vi "Plotter_Plot_Core.vi"(7 "Plot Parameters":T1[](array[typedef]), 8 "error in (no error)":errorcluster, 9 "Refresh interval (ms)":u32, 10 "Commands":T2, 11 "XY Graph":refnum<vi>) -> (0 "error out":errorcluster)   [LabVIEW 2017]
uses:
  Controls/Plotter_UI_Plot_Commands.ctl
  Controls/Plotter_Plot_Parameter_and_Timestamp.ctl
  Controls/Plotter_Plot.ctl
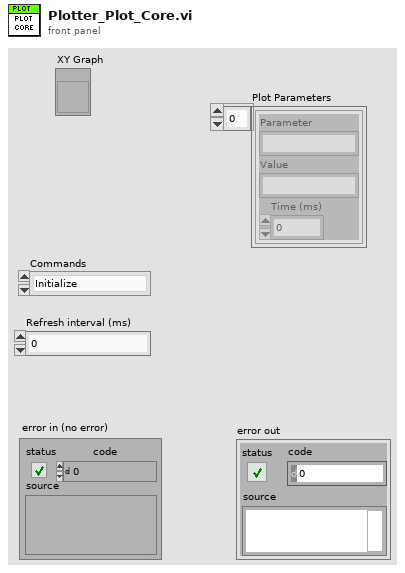
[diagram p1: front panel]
types:
  T1 = typedef "Plotter_Plot_Parameter_and_Timestamp.ctl" = cluster{"Parameter":string, "Value":string, "Time (ms)":u32}
  T2 = typedef "Plotter_UI_Plot_Commands.ctl" = enum16{"Initialize", "Update", "Clear"}
  T3 = typedef "Plotter_Plot.ctl" = cluster{"Time (ms)":dbl[], "Values":dbl[]}
  T4 = cluster{"Parameter name":string, "Samples":dbl[], "Time (ms)":dbl[]}[]
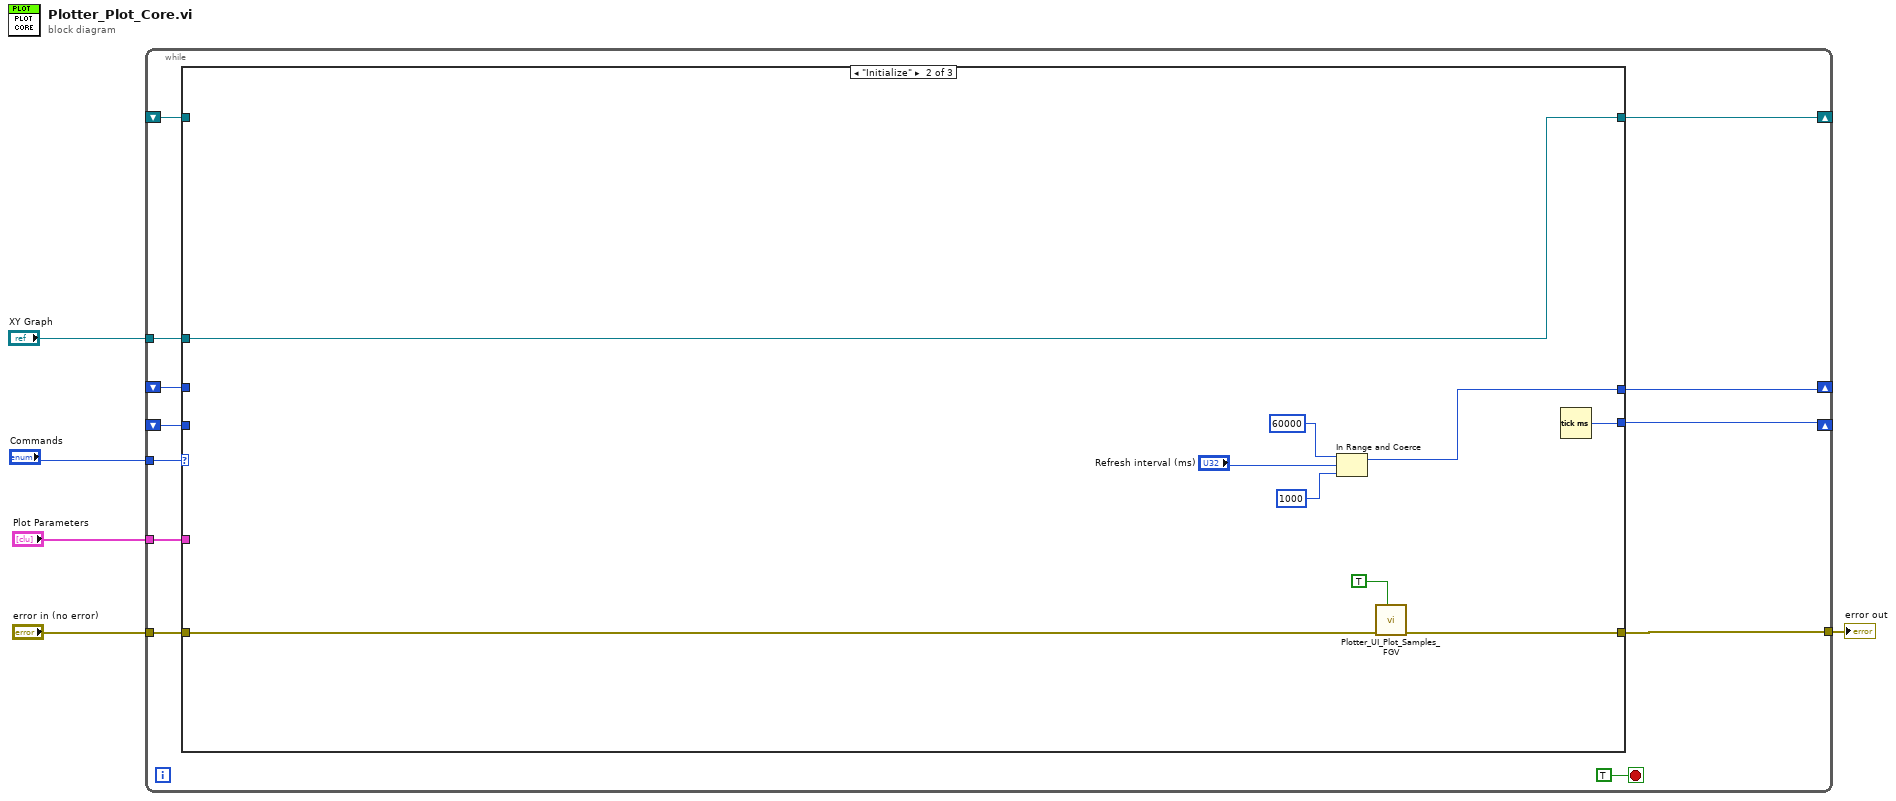
[diagram p0: block diagram]
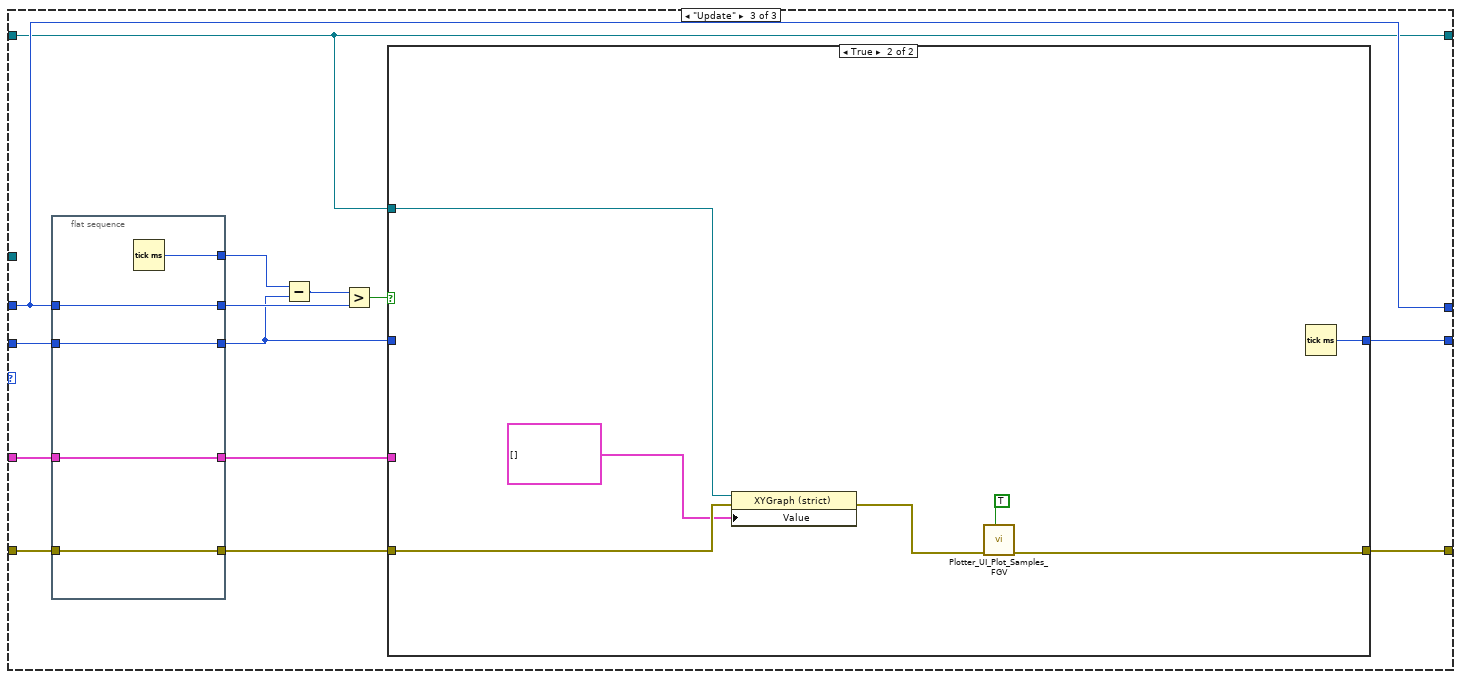
[diagram p3: hidden frame]
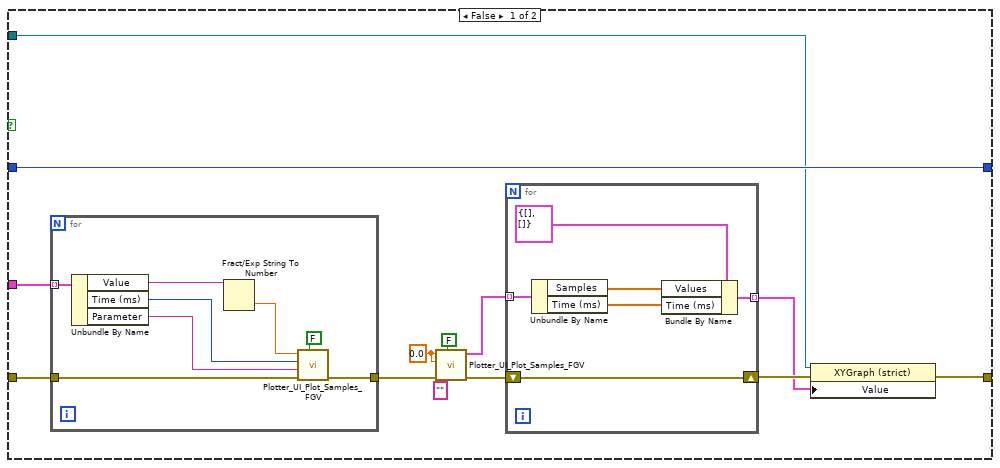
[diagram p4: hidden frame]
diagram:
  n1 = while {
    tunnel: "XY Graph" -> [w15]
    tunnel: "error in (no error)" -> [w12]
    tunnel: "Commands" -> [w16]
    shift-right: [w14] -> _
    shift-left: _ -> [w13]
    tunnel: [w11] -> w1
    shift-right: [w10] -> _
    shift-left: _ -> [w8]
    shift-right: [w9] -> _
    shift-left: _ -> [w7]
    tunnel: "Plot Parameters" -> [w6]
    stop <- TRUE stop-if-true
    n2 = case shown="\"Initialize\"" w16 {
      tunnel: w15 -> [_ w30 _]
      tunnel: [w21 w30 w31] -> w14
      tunnel: w13 -> [w21 _ w31]
      tunnel: w12 -> [w20 w24 w44]
      tunnel: [w20 w23 w34] -> w11
      tunnel: [w19 w25 w39] -> w10
      tunnel: [w18 w29 w37] -> w9
      tunnel: w8 -> [w19 _ w39]
      tunnel: w7 -> [w18 _ w43]
      tunnel: w6 -> [_ _ w33]
      frame Default {
      }
      frame "Initialize" {
        n3 = In Range and Coerce(upper limit=u32 60000, x="Refresh interval (ms)", lower limit=u32 1000) -> (coerced(x)=w25:u32)  [unwired: 1 out]
        n4 = call "Plotter_UI_Plot_Samples_FGV.vi"("Initialize ?"=TRUE, "error in (no error)"=w24) -> ("error out"=w23:errorcluster)  [unwired: 8 in, 1 out]
        n5 = Tick Count (ms)() -> (millisecond timer value=w29:u32)
      }
      frame "Update" {
        n6 = flat-sequence {
          tunnel: w44 -> [w83]
          tunnel: [w83] -> w35
          tunnel: w43 -> [w82]
          tunnel: [w82] -> w36
          tunnel: [w81] -> w42
          tunnel: w39 -> [w80]
          tunnel: [w80] -> w40
          tunnel: w33 -> [w79]
          tunnel: [w79] -> w32
          frame #0 {
            n7 = Tick Count (ms)() -> (millisecond timer value=w81:u32)
          }
        }
        n8 = Subtract(x=w42, y=w36) -> (x-y=w41:u32)
        n9 = Greater?(x=w41, y=w40) -> (0:w38:bool)
        n10 = case shown="True" w38 {
          tunnel: [w57 w78] -> w37
          tunnel: w36 -> [w57 _]
          tunnel: w35 -> [w56 w77]
          tunnel: [w47 w73] -> w34
          tunnel: w32 -> [w55 _]
          tunnel: w31 -> [w46 w76]
          frame False {
            w52 = 0.0 ("Value")
            n11 = for {
              tunnel: w56 -> [w71]
              tunnel: w55 -> [w69] mode=indexing
              tunnel: [w64] -> w54
              n12 = Unbundle By Name(w69) -> ("Value"=w68:string, "Time (ms)"=w66:u32, "Parameter"=w65:string)
              n13 = Fract/Exp String To Number(string=w68) -> (number=w67:dbl)  [unwired: 3 in, 1 out]
              n14 = call "Plotter_UI_Plot_Samples_FGV.vi"("Initialize ?"=FALSE, "error in (no error)"=w71, "Parameter name"=w65, "Time (ms)"=w66, "Value"=w67) -> ("error out"=w64:errorcluster)  [unwired: 5 in, 1 out]
            }
            n15 = call "Plotter_UI_Plot_Samples_FGV.vi"("Initialize ?"=FALSE, "error in (no error)"=w54, "Parameter name"="", "Time (ms)"=w52, "Value"=w52) -> ("error out"=w49:errorcluster, "Samples & timestamp"=w50:T4)  [unwired: 5 in]
            n16 = for {
              tunnel: w50 -> [w62] mode=indexing
              shift-right: [w63] -> w48
              shift-left: w49 -> [w63]
              tunnel: [w58] -> w45 mode=indexing
              n17 = Unbundle By Name(w62) -> ("Samples"=w60:dbl[], "Time (ms)"=w59:dbl[])
              n18 = Bundle By Name(cluster=T3 {"Time (ms)"=[], "Values"=[]} ("output cluster"), "Values"=w60, "Time (ms)"=w59) -> (w58:T3)
            }
            n19 = property class="XYGraph (strict)"(reference=w46, error in=w48, "Value"=w45) -> (error out=w47:errorcluster)  [unwired: 1 out]
          }
          frame True {
            n20 = property class="XYGraph (strict)"(reference=w76, error in=w77, "Value"=cluster{"Time (ms)":dbl[], "Values":dbl[]}[] []) -> (error out=w74:errorcluster)  [unwired: 1 out]
            n21 = call "Plotter_UI_Plot_Samples_FGV.vi"("Initialize ?"=TRUE, "error in (no error)"=w74) -> ("error out"=w73:errorcluster)  [unwired: 8 in, 1 out]
            n22 = Tick Count (ms)() -> (millisecond timer value=w78:u32)
          }
        }
      }
    }
  }
  "error out" <- w1
